vi "Digital1GHzOszi-Host.vi"() -> ()   [LabVIEW 2012]
uses:
  <vilib>/FPGAPlugInAG/PXIe-7962R/niLvFpga_Open_PXIe-7962R.vi
  <vilib>/rvi/interface/common/dynamic/niFpgaDynamicAddResources.vi
  <vilib>/Utility/error.llb/Error Cluster From Error Code.vi
  <vilib>/rvi/errors/niLvFpgaAdjustHostInterfaceError.vi
  <vilib>/FPGAPlugInAG/Dynamic/niLvFpga_Close_Dynamic.vi
  <vilib>/rvi/interface/nirviOpenFPGA/nirviOpenFPGA.xnode
  FPGA Bitfiles/DigitalOszi_PXIe-7962R.lvbitx
  FPGAVIs/DigitalOszi_PXIe-7962R.vi
  <vilib>/rvi/interface/nirviReadWriteControl/nirviReadWriteControl.xnode
  <vilib>/rvi/interface/nirviMethod/nirviMethod.xnode
  <vilib>/rvi/interface/nirviCloseFPGA/nirviCloseFPGA.xnode
  <vilib>/rvi/interface/Simulation/niFpgaSimulationCallBeginRW.vi
  NiFpgaLv.dll
  <vilib>/FPGAPlugInAG/Dynamic/niLvFpga_ReadFifo_Dynamic.vi
  <vilib>/rvi/errors/niLvFpgaMergeErrorWithErrorCode.vi
panel:
  out "effective MBit/s":dbl
  out "Read rate (Hz)":dbl
  out "Elements Remaining":u32
  out "ToHost Overflow":bool
  out "Interloop Timed Out?":bool
  out "Graph":i16[](graph)
  in  "Quit":bool
  in  "Commit&Start":bool
  in  "Clock Freq (Hz)":dbl=100000000.0 format="%#_6p"
  in  "error in":errorcluster
  # "NI 6587 I/O Module Configuration"
  # "(reading U64, but only 60 bits with data)"
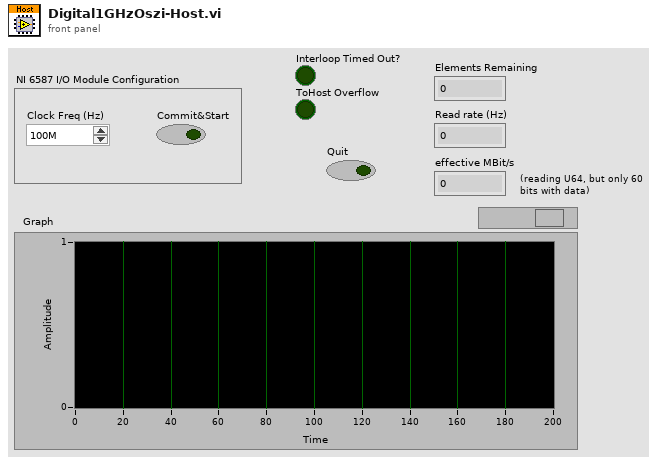
[diagram p1: front panel]
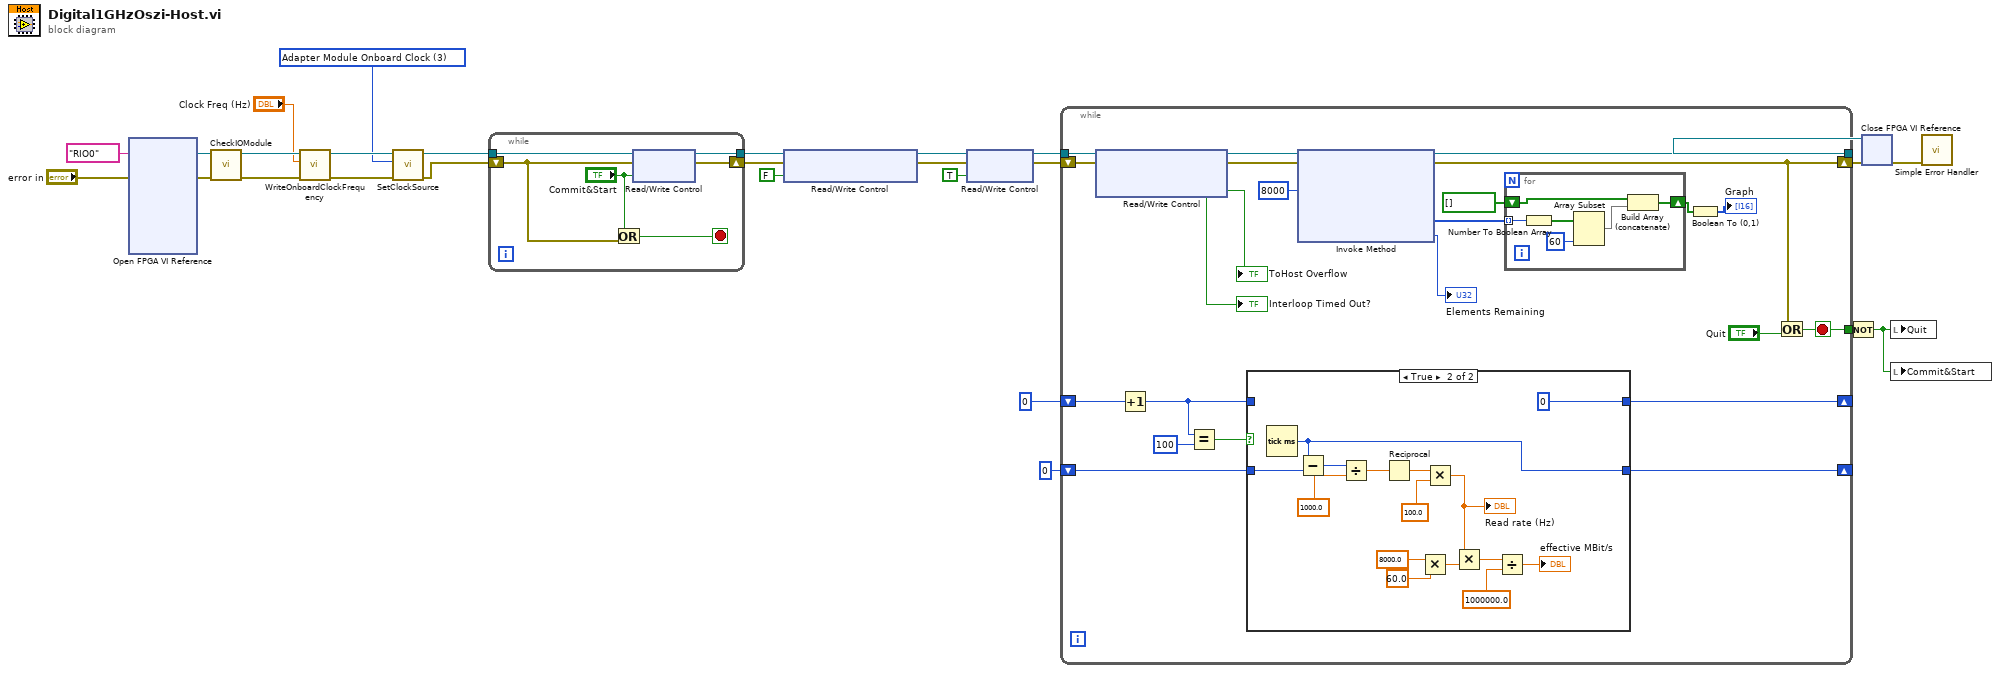
[diagram p0: block diagram]
diagram:
  w3 = u8 3 items=["Tristate"=0, "Sync Clock (PXIe only)"=2, "Adapter Module Onboard Clock"=3, "Strobe from Crosspoint Switch"=4, "Strobe Bypass"=5] ("Clock Source")
  n1 = xnode "Open FPGA VI Reference"("error in"="error in", "resource name"=tag "RIO0") -> ("FPGA VI Reference Out"=w9:refnum<k20>, "error out"=w10:errorcluster)
  n2 = call "CheckIOModule.vi"("error in (no error)"=w10, "FPGA VI Reference In"=w9) -> ("error out"=w8:errorcluster, "FPGA VI Reference Out"=w7:refnum<k20>)  [unwired: 8 in]
  n3 = call "WriteOnboardClockFrequency.vi"("error in (no error)"=w8, "Onboard clock frequency"="Clock Freq (Hz)", "FPGA VI Reference In"=w7) -> ("error out"=w5:errorcluster, "FPGA VI Reference Out"=w4:refnum<k20>)  [unwired: 7 in]
  n4 = call "SetClockSource.vi"("error in (no error)"=w5, "Clock Source"=w3, "FPGA VI Reference In"=w4) -> ("error out"=w1:errorcluster, "FPGA VI Reference Out"=w2:refnum<k20>)  [unwired: 7 in]
  n5 = while {
    tunnel: w2 -> [w33]
    shift-right: [w32] -> w25
    shift-left: w1 -> [w29]
    tunnel: [w31] -> w24
    stop <- w28 stop-if-true
    n6 = Or(x="Commit&Start", y=w29) -> (x .or. y?=w28:bool)
    n7 = xnode "Read/Write Control"("FPGA VI Reference In"=w33, "error in"=w29, "Commit"="Commit&Start") -> ("FPGA VI Reference Out"=w31:refnum<k20>, "error out"=w32:errorcluster)
  }
  n8 = xnode "Read/Write Control"("FPGA VI Reference In"=w24, "error in"=w25, "IO Module\\Acq_Reset"=FALSE ("IO Module\\Acq_Reset")) -> ("FPGA VI Reference Out"=w18:refnum<k20>, "error out"=w19:errorcluster)
  n9 = xnode "Read/Write Control"("FPGA VI Reference In"=w18, "error in"=w19, "Start Acq"=TRUE) -> ("FPGA VI Reference Out"=w16:refnum<k20>, "error out"=w17:errorcluster)
  n10 = while {
    tunnel: w16 -> [w46]
    shift-right: [w49] -> w21
    shift-left: w17 -> [w45]
    tunnel: [w50] -> w22
    shift-right: [w53] -> _
    shift-left: u32 0 ("millisecond timer value") -> [w52]
    tunnel: [w51] -> w13
    shift-right: [w38] -> _
    shift-left: 0 -> [w42]
    stop <- w51 stop-if-true
    n11 = xnode "Read/Write Control"("FPGA VI Reference In"=w46, "error in"=w45) -> ("FPGA VI Reference Out"=w44:refnum<k20>, "error out"=w43:errorcluster, "Interloop Timed Out?"=→"Interloop Timed Out?":bool, "ToHost overflow"=→"ToHost Overflow":bool)
    n12 = Increment(x=w42) -> (x+1=w39:i32)
    n13 = Equal?(x=w39, y=100) -> (x = y?=w40:bool)
    n14 = case shown="True" w40 {
      tunnel: [w64 w79] -> w53
      tunnel: w52 -> [w64 w78]
      tunnel: w39 -> [w63 _]
      tunnel: [w63 0] -> w38
      frame False {
      }
      frame True {
        n15 = Tick Count (ms)() -> (millisecond timer value=w79:u32)
        n16 = Subtract(x=w79, y=w78) -> (x-y=w77:u32)
        n17 = Divide(x=w77, y=1000.0) -> (x/y=w75:dbl)
        n18 = Reciprocal(x=w75) -> (1/x=w74:dbl)
        n19 = Multiply(x=8000.0, y=60.0) -> (x*y=w68:dbl)
        n20 = Multiply(x=w74, y=100.0) -> (x*y=w71:dbl)
        "Read rate (Hz)" <- w71
        n21 = Multiply(x=w71, y=w68) -> (x*y=w67:dbl)
        n22 = Divide(x=w67, y=1000000.0) -> (x/y=→"effective MBit/s":dbl)
      }
    }
    n23 = xnode "Invoke Method"("FPGA VI Reference In"=w44, "error in"=w43, "Number of Elements"=u32 8000) -> ("FPGA VI Reference Out"=w50:refnum<k20>, "error out"=w49:errorcluster, "Data"=w37:u64[], "Elements Remaining"=→"Elements Remaining":u32)  [unwired: 1 in]
    n24 = for {
      tunnel: w37 -> [w62] mode=indexing
      shift-right: [w58] -> w35
      shift-left: bool[] [] -> [w57]
      n25 = Number To Boolean Array(number=w62) -> (Boolean array=w61:bool[])
      n26 = Array Subset(array=w61, length=60) -> (w59:bool[])  [unwired: 1 in]
      n27 = Build Array (concatenate)(w57, w59) -> (w58:bool[])
    }
    n28 = Boolean To (0,1)(Boolean=w35) -> (0, 1=→"Graph":i16[])
    n29 = Or(x=w49, y="Quit") -> (x .or. y?=w51:bool)
  }
  n30 = Not(x=w13) -> (.not. x?=w12:bool)
  n31 = xnode "Close FPGA VI Reference"("FPGA VI Reference In"=w22, "error in"=w21) -> ("error out"=w20:errorcluster)
  n32 = local write "Quit"(w12) -> ()
  n33 = local write "Commit&Start"(w12) -> ()
  n34 = call <vilib>:"Simple Error Handler.vi"("error in (no error)"=w20) -> ()  [unwired: 4 in, 5 out]
